vi "吸收概率设置.vi"(2 "错误输入（无错误）":errorcluster, 3 "衰减":dbl, 4 "VISA资源名称":refnum<visa-resource-name>) -> (0 "错误输出":errorcluster, 1 "VISA资源名称输出":refnum<visa-resource-name>)   [LabVIEW 2014]
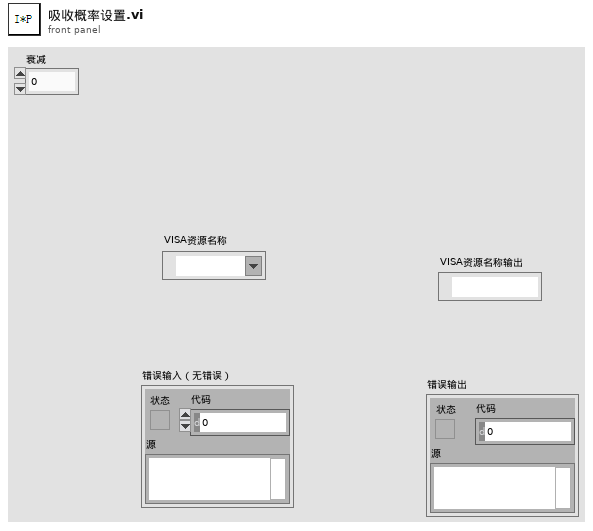
[diagram p1: front panel]
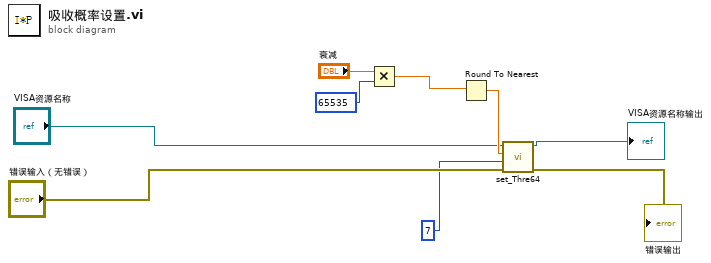
[diagram p0: block diagram]
diagram:
  n1 = Multiply(x="衰减", y=u16 65535) -> (x*y=w1:dbl)
  n2 = Round To Nearest(number=w1) -> (nearest integer value=w6:dbl)
  n3 = call "set_Thre64.vi"("错误输入（无错误）"="错误输入（无错误）", "命令"=7, "数字"=w6, "VISA资源名称"="VISA资源名称") -> ("错误输出"=→"错误输出":errorcluster, "VISA资源名称输出"=→"VISA资源名称输出":refnum<visa-resource-name>)  [unwired: 6 in]
